vi "CRYRound Zero Padder.vi"(10 "Significant Digit":u8=2, 11 "Vector in":dbl[](array[numeric])) -> (2 "Zero Padding Number":i32, 3 "Zero Padder Vector out":dbl[](array[numeric]))   [LabVIEW 2013]
panel:
  # "Significant Zero Padding."
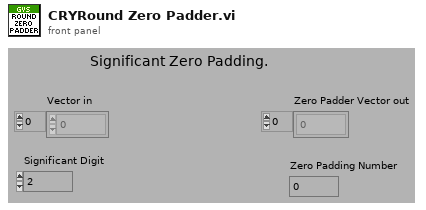
[diagram p1: front panel]
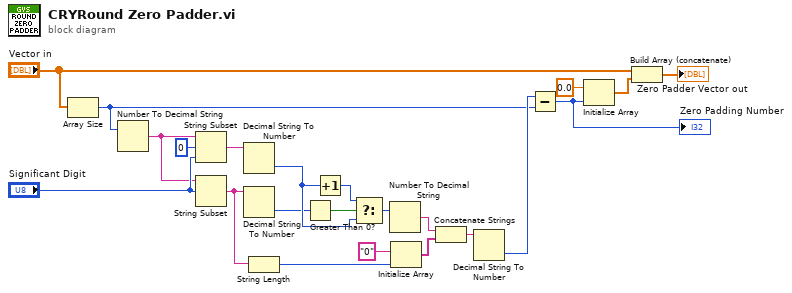
[diagram p0: block diagram]
diagram:
  n1 = Array Size(array="Vector in") -> (size(s)=w2:i32)
  n2 = Number To Decimal String(number=w2) -> (decimal integer string=w18:string)  [unwired: 1 in]
  n3 = String Subset(string=w18, offset (0)=0, length (rest)="Significant Digit") -> (substring=w13:string)
  n4 = String Subset(string=w18, offset (0)="Significant Digit") -> (substring=w16:string)  [unwired: 1 in]
  n5 = Decimal String To Number(string=w13) -> (number=w12:i32)  [unwired: 2 in, 1 out]
  n6 = Decimal String To Number(string=w16) -> (number=w4:i32)  [unwired: 2 in, 1 out]
  n7 = String Length(string=w16) -> (length=w15:i32)
  n8 = Greater Than 0?(x=w4) -> (x > 0?=w20:bool)
  n9 = Increment(x=w12) -> (x+1=w19:i32)
  n10 = Select(t=w19, s=w20, f=w12) -> (s? t:f=w11:i32)
  n11 = Number To Decimal String(number=w11) -> (decimal integer string=w10:string)  [unwired: 1 in]
  n12 = Initialize Array("0" ("substring"), w15) -> (w14:string[])
  n13 = Concatenate Strings(w10, w14) -> (w9:string)
  n14 = Decimal String To Number(string=w9) -> (number=w7:i32)  [unwired: 2 in, 1 out]
  n15 = Subtract(x=w7, y=w2) -> (x-y=w1:i32)
  "Zero Padding Number" <- w1
  n16 = Initialize Array(0.0 ("Numeric 2"), w1) -> (w5:dbl[])
  n17 = Build Array (concatenate)("Vector in", w5) -> (→"Zero Padder Vector out":dbl[])
